vi "Get VI Ref.vi"(8 "error in (no error)":errorcluster, 11 "Test Helper 1 in":refnum<class "Test Helper 1.lvclass">) -> (0 "error out":errorcluster, 1 "VI Clone Name":string, 2 "Static VI Ref":refnum<vi>, 3 "Test Helper 1 out":refnum<class "Test Helper 1.lvclass">)   [LabVIEW 2019, in "Test Helper 1.lvclass"]
uses:
  Test Helper 1.lvclass
  <vilib>/JKI/JKI SMO/SMO/SMO.lvclass
  C:/Program Files (x86)/National Instruments/LabVIEW 2020/vi.lib/JKI/JKI SMO/SMO/SMO.lvclass
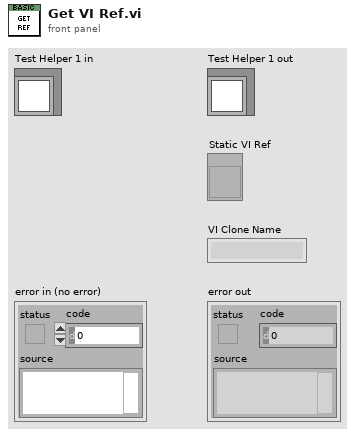
[diagram p1: front panel]
types:
  T1 = typedef "SMO.lvclass/RegisteredProcessData--Cluster.ctl" = cluster{"Name":string, "Static VI Ref":refnum<vi>, "Running":bool, "NotifierRef":u32}
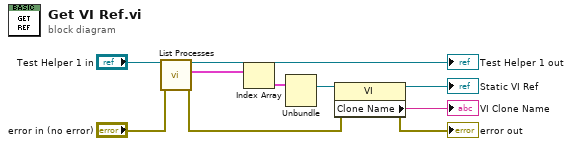
[diagram p0: block diagram]
diagram:
  n1 = call <vilib>:"List Processes.vi"("error in (no error)"="error in (no error)", "SMO"="Test Helper 1 in") -> ("error out"=w2:errorcluster, "Registered Processes"=w9:T1[], "SMO out"=→"Test Helper 1 out":refnum<class "Test Helper 1.lvclass">)  [unwired: 7 in]
  n2 = Index Array(array=w9) -> (element=w8:T1)  [unwired: 1 in]
  n3 = Unbundle(w8) -> ("Static VI Ref"=w5:refnum<vi>)  [unwired: 3 out]
  n4 = property class="VI"(reference=w5, error in=w2) -> (reference out=→"Static VI Ref":refnum<vi>, error out=→"error out":errorcluster, "Clone Name"=→"VI Clone Name":string)
